vi "get-data.vi"(8 "error in (no error)":errorcluster, 11 "tempy in":refnum<class "array-in-a-cluster.lvclass">) -> (0 "error out":errorcluster, 2 "Cluster.Array":bool[](array[boolean]), 3 "tempy out":refnum<class "array-in-a-cluster.lvclass">)   [LabVIEW 2020, in "TEST - JKI JSON Object Serialization.lvlib" / "array-in-a-cluster.lvclass"]
uses:
  array-in-a-cluster.lvclass
  array-in-a-cluster.lvclass/array-in-a-cluster.ctl
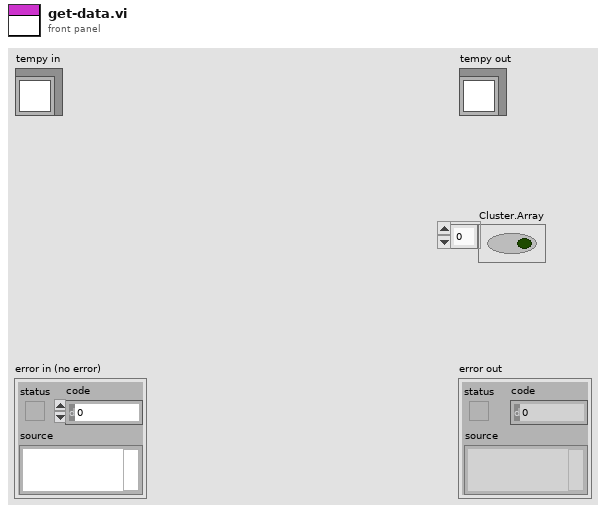
[diagram p1: front panel]
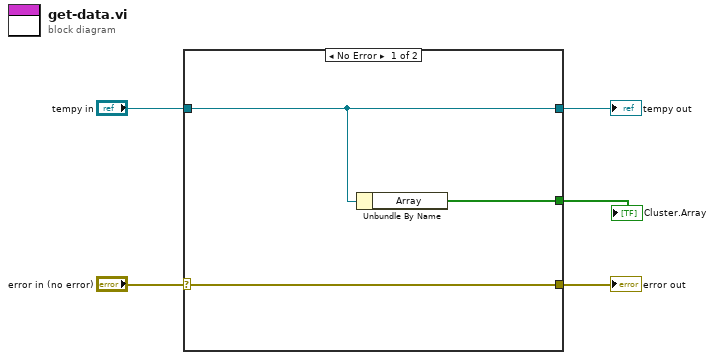
[diagram p0: block diagram]
diagram:
  n1 = case shown="No Error" "error in (no error)" {
    selector: "error in (no error)" -> [w8 w10]
    tunnel: [w8 w10] -> w4
    tunnel: [w7 w9] -> w2
    tunnel: "tempy in" -> [w7 w9]
    tunnel: [w6 _] -> w1
    frame No Error {
      n2 = Unbundle By Name(w7) -> ("Array"=w6:bool[])
    }
    frame Error {
    }
  }
  "error out" <- w4
  "tempy out" <- w2
  "Cluster.Array" <- w1
